vi "Configure Current Limit.vi"(8 "error in (no error)":errorcluster, 9 "Current Limit (0.0 Amps)":dbl format="%.2p", 11 "VISA resource name":refnum<visa-resource-name>) -> (0 "error out":errorcluster, 3 "VISA resource name out":refnum<visa-resource-name>)   [LabVIEW 2022 SP3, in "Agilent E364X Series.lvlib"]
doc: "This VI configures the current limit. You specify the output current limit value and the behavior of the power supply when the output current is greater than or equal to that value.\n\nNotes:\n\n(1) The only behavior currently available with the HP E364xA series is to regulate the current when the limit is passed or reached."
uses:
  Agilent E364X Series.lvlib
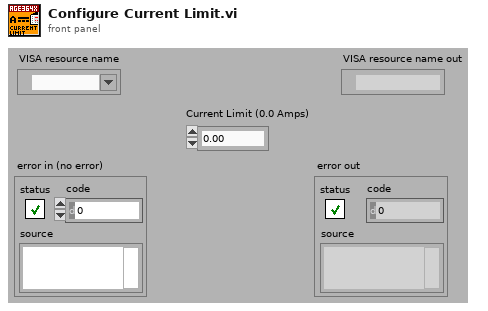
[diagram p1: front panel]
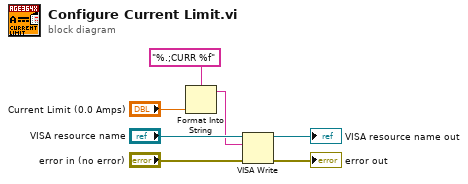
[diagram p0: block diagram]
diagram:
  n1 = Format Into String(format string="%.;CURR %f", "Current Limit (0.0 Amps)") -> (resulting string=w1:string)  [unwired: 2 in, 1 out]
  n2 = VISA Write(VISA resource name="VISA resource name", write buffer=w1, error in (no error)="error in (no error)") -> (VISA resource name out=→"VISA resource name out":refnum<visa-resource-name>, error out=→"error out":errorcluster)  [unwired: 1 out]
